vi "Collate 32Ch Port.vi"(9 "Indices":i32[](array[numeric]), 10 "U32 Port":u32, 11 "Values in":dbl[](array[numeric])) -> (3 "Values":dbl[](array[numeric]))   [LabVIEW 2020, in "VolatusDAQ.lvlib" / "DAQmxDI.lvclass"]
uses:
  DAQmxDI.lvclass
  DAQmxDI.lvclass/DAQmxDI.ctl
  lv-vecto/Vecto/Vecto.lvlib
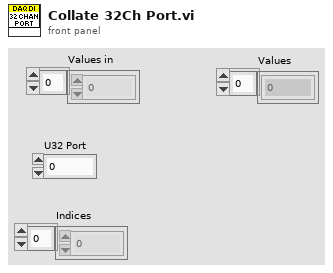
[diagram p1: front panel]
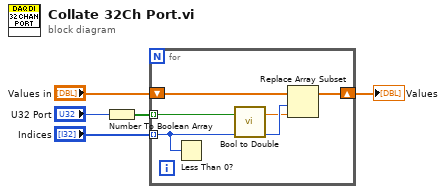
[diagram p0: block diagram]
diagram:
  n1 = Number To Boolean Array(number="U32 Port") -> (Boolean array=w5:bool[])
  n2 = for {
    tunnel: w5 -> [w10] mode=indexing
    tunnel: "Indices" -> [w7] mode=indexing
    shift-right: [w8] -> w1
    shift-left: "Values in" -> [w9]
    n3 = Less Than 0?(x=w7) -> ()  [unwired: 1 out]
    n4 = call "Bool to Double.vi"("Bool"=w10) -> ("Double"=w6:dbl)  [unwired: 2 in]
    n5 = Replace Array Subset(array=w9, new element=w6, index=w7) -> (w8:dbl[])
  }
  "Values" <- w1
